vi "GetFiles.vi"(8 "error in (no error)":errorcluster, 11 "Python":T1) -> (0 "error out":errorcluster, 3 "all files":string[](array[string]))   [LabVIEW 2022 SP3]
uses:
  PythonCtrl.ctl
  Processors.ctl
panel:
  out "Console":string
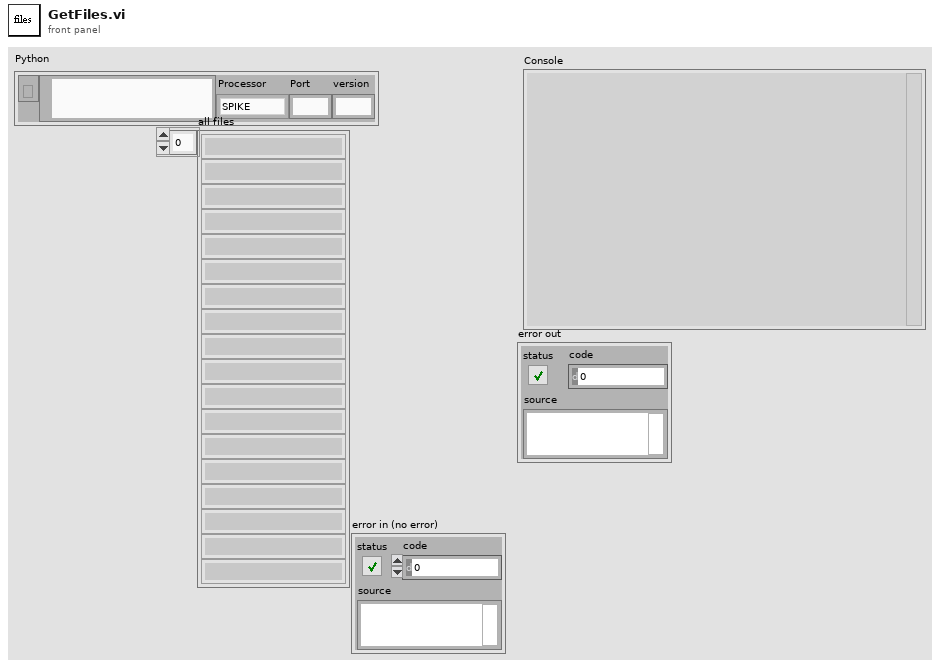
[diagram p1: front panel]
types:
  T1 = typedef "PythonCtrl.ctl" = cluster{"session":refnum<k35>, "PyPath":path, "Processor":T2, "Port":string, "version":string}
  T2 = typedef "Processors.ctl" = enum16{"SPIKE", "Pi", "Pi_ssh", "OpenMV", "Dunio"}
  T3 = enum16{"read", "write pause", "write port", "write path", "write all"}
  T4 = enum8{"Enabled", "Disabled", "Disabled and Grayed Out"}
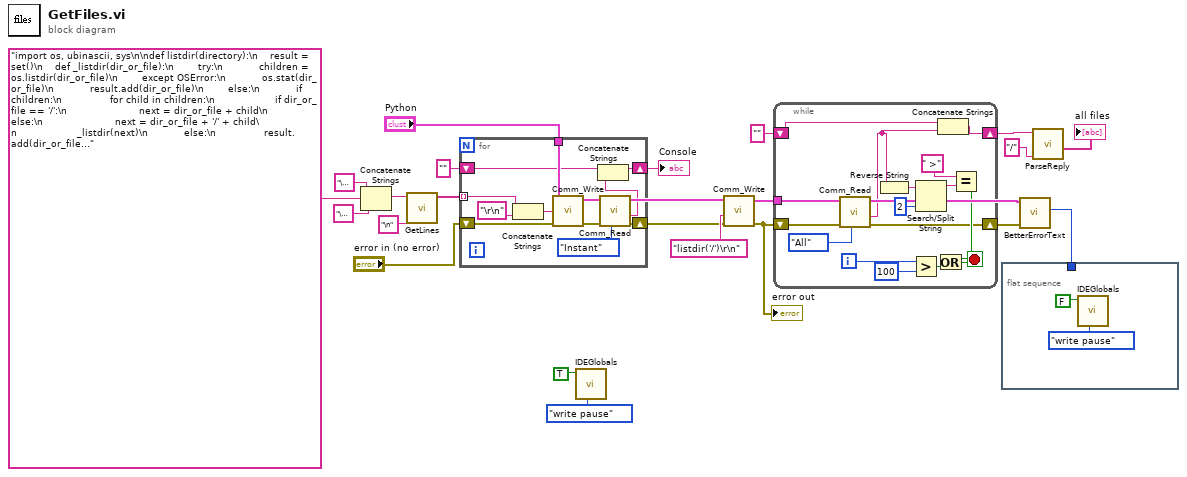
[diagram p0: block diagram]
diagram:
  n1 = Concatenate Strings("\u0005" ("string"), "import os, ubinascii, sys\n\ndef listdir(directory):\n    result = set()\n    def _listdir(dir_or_file):\n        try:\n            children = os.listdir(dir_or_file)\n        except OSError:\n            os.stat(dir_or_file)\n            result.add(dir_or_file)\n        else:\n            if children:\n                for child in children:\n                    if dir_or_file == '/':\n                        next = dir_or_file + child\n                    else:\n                        next = dir_or_file + '/' + child\n                    _listdir(next)\n            else:\n                result.add(dir_or_file)\n    _listdir(directory)\n    return sorted(result)\n\ndef readfile(file):\n    with open(file, 'rb') as infile:\n        while True:\n            result = infile.read(32)\n            if result == b'':\n                break\n            len = sys.stdout.write(ubinascii.hexlify(result))\n\n" ("function name"), "\u0004" ("string")) -> (w12:string)
  n2 = call "GetLines.vi"("delimiter"="\n" ("function name"), "String"=w12) -> ("Array"=w9:string[])  [unwired: 9 in]
  n3 = for {
    tunnel: "Python" -> [w28]
    shift-right: [w29] -> w13
    shift-left: "error in (no error)" -> [w32]
    tunnel: w9 -> [w27] mode=indexing
    shift-right: [w23] -> w10
    shift-left: "" -> [w25]
    n4 = Concatenate Strings(w27, "\r\n" ("function name")) -> (w26:string)
    n5 = call "Comm_Write.vi"("error in (no error)"=w32, "Text to write"=w26, "Python"=w28) -> ("error out"=w31:errorcluster)  [unwired: 7 in, 1 out]
    n6 = call "Comm_Read.vi"("Task"=enum16{"Instant", "All", "AllFast", "Params"}."Instant", "error in (no error)"=w31, "Python"=w28) -> ("error out"=w29:errorcluster, "Text read"=w24:string)  [unwired: 7 in]
    n7 = Concatenate Strings(w25, w24) -> (w23:string)
  }
  "Console" <- w10
  n8 = call "IDEGlobals.vi"("task"=T3."write pause", "pause?"=TRUE) -> ()  [unwired: 7 in, 3 out]
  n9 = call "Comm_Write.vi"("error in (no error)"=w13, "Text to write"="listdir('/')\r\n" ("function name"), "Python"="Python") -> ("error out"=w18:errorcluster)  [unwired: 7 in, 1 out]
  "error out" <- w18
  n10 = while {
    tunnel: "Python" -> [w47]
    shift-right: [w34] -> w20
    shift-left: "" ("Text read") -> [w36]
    shift-right: [w33] -> w5
    shift-left: w18 -> [w46]
    i -> [w45]
    stop <- w42 stop-if-true
    n11 = call "Comm_Read.vi"("Task"=enum16{"Instant", "All", "AllFast"}."All", "error in (no error)"=w46, "Python"=w47) -> ("error out"=w33:errorcluster, "Text read"=w35:string)  [unwired: 7 in]
    n12 = Reverse String(1:w35) -> (0:w41:string)
    n13 = Greater?(x=w45, y=100) -> (0:w43:bool)
    n14 = Search/Split String(string=w41, offset (0)=2) -> (substring before match=w39:string)  [unwired: 1 in, 2 out]
    n15 = Concatenate Strings(w36, w35) -> (w34:string)
    n16 = Equal?(x=" >", y=w39) -> (x = y?=w37:bool)
    n17 = Or(x=w37, y=w43) -> (x .or. y?=w42:bool)
  }
  n18 = flat-sequence {
    tunnel: w1 -> [_]
    frame #0 {
      n19 = call "IDEGlobals.vi"("task"=T3."write pause", "pause?"=FALSE) -> ()  [unwired: 7 in, 3 out]
    }
  }
  n20 = call "BetterErrorText.vi"("error in (no error)"=w5, "Python"="Python") -> ("Disabled"=w1:T4)  [unwired: 8 in, 1 out]
  n21 = call "ParseReply.vi"("Parent"="/" ("trimmed string"), "Console"=w20) -> ("PythonFiles"=→"all files":string[])  [unwired: 7 in, 2 out]
